vi "20150713Ultrasonic distance measurement(LINX).vi"() -> ()   [LabVIEW 2013]
uses:
  <vilib>/MakerHub/LINX/Public/Sensors/Ultrasonic/Ultrasonic.lvlib
  <vilib>/MakerHub/LINX/LMH-LINX.lvlib
panel:
  out "Initialize OK?":bool
  out "Error Out":errorcluster
  in  "Error In":errorcluster
  out "Centimeters":dbl
  in  "stop":bool
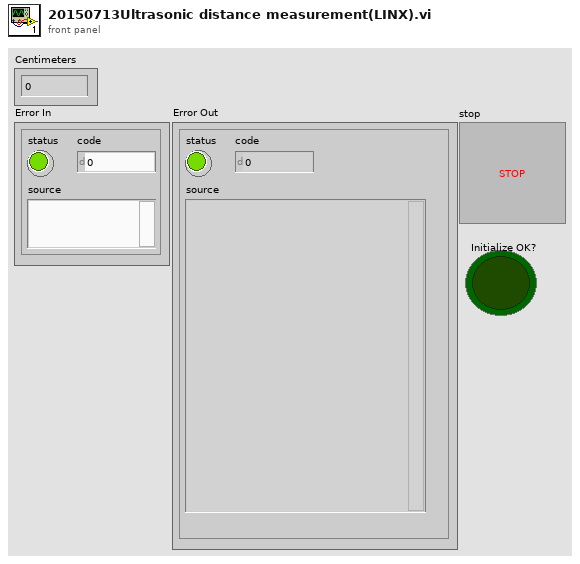
[diagram p1: front panel]
types:
  T1 = typedef "LMH-LINX.lvlib/LINX Ref.ctl" = cluster{"Platform":T2, "Interface":T3, "LINX Device Config":T4}
  T2 = typedef "LMH-LINX.lvlib/Platform.ctl" = enum16{"LINX", "myRIO"}
  T3 = typedef "LMH-LINX.lvlib/Interface.ctl" = enum16{"Serial", "TCP"}
  T4 = typedef "LMH-LINX.lvlib/Device.lvlib/LINX Device Config.ctl" = cluster{"Interface":T3, "COM Port":refnum<visa-resource-name>, "TCP Configuration":T5, "Device Family":u8, "Device ID":u8, "Device Name":string, "TCP Ref":refnum<k5>, "Channels":T6}
  T5 = typedef "LMH-LINX.lvlib/Device.lvlib/TCP Config.ctl" = cluster{"IP Address":string, "Port":u16}
  T6 = typedef "LMH-LINX.lvlib/Channels.ctl" = cluster{"DI":u8[], "DO":u8[], "AI":u8[], "AO":u8[], "PWM":u8[], "QE":u8[], "UART":u8[], "I2C 2":u8[], "SPI":u8[], "CAN":u8[], "Servo":u8[], "AI Ref (V)":dbl, "AO Ref (V)":dbl, "AO Resolution (Bits)":u8}
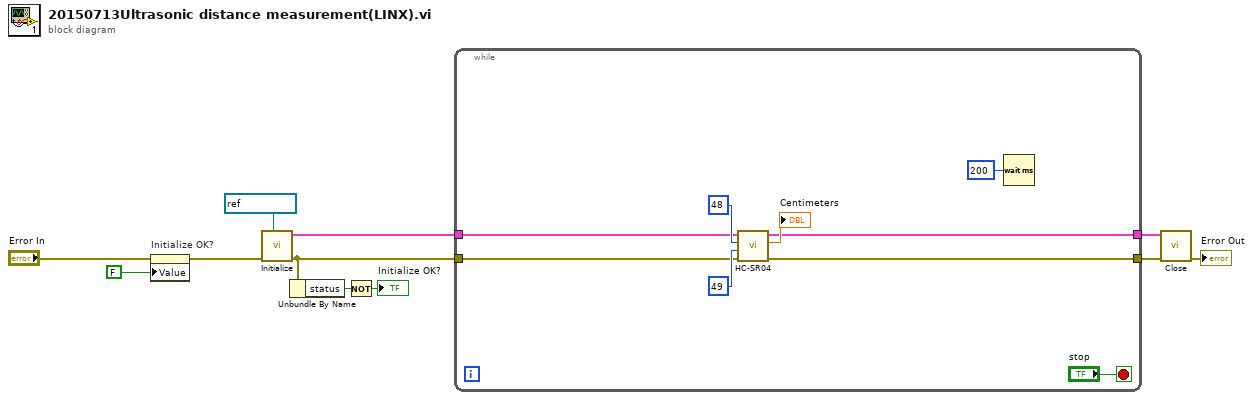
[diagram p0: block diagram]
diagram:
  n1 = property on="Initialize OK?" class="Bool (strict)"(error in="Error In", "Value"=FALSE ("Initialize OK?")) -> (error out=w1:errorcluster)  [unwired: 1 in, 1 out]
  n2 = call <vilib>:"Initialize.vi"("Serial Port"=refnum<visa-resource-name> "COM10", "Error In"=w1) -> ("Error Out"=w6:errorcluster, "LINX Ref"=w7:T1)  [unwired: 7 in, 1 out]
  n3 = Unbundle By Name(w6) -> ("status"=w5:bool)
  n4 = Not(x=w5) -> (.not. x?=→"Initialize OK?":bool)
  n5 = while {
    tunnel: [w16] -> w11
    tunnel: [w15] -> w10
    tunnel: w7 -> [w14]
    tunnel: w6 -> [w13]
    stop <- "stop" stop-if-true
    n6 = call <vilib>:"HC-SR04.vi"("Error In"=w13, "Echo Pin (DI)"=u8 49, "Trig"=u8 48, "LINX Resource"=w14) -> ("Error Out"=w15:errorcluster, "Centimeters"=→"Centimeters":dbl, "LINX Resource"=w16:T1)  [unwired: 4 in, 1 out]
    n7 = Wait (ms)(milliseconds to wait=u32 200) -> ()  [unwired: 1 out]
  }
  n8 = call <vilib>:"Close.vi"("Error In"=w10, "LINX Resource"=w11) -> ("Error Out"=→"Error Out":errorcluster)  [unwired: 8 in, 1 out]
